vi "getCost.vi"(8 "error in (no error)":errorcluster, 11 "Espresso in":refnum<class "Espresso.lvclass">) -> (0 "error out":errorcluster, 2 "cost":dbl, 3 "Espresso out":refnum<class "Espresso.lvclass">)   [LabVIEW 2018, in "Espresso.lvclass"]
uses:
  Espresso.lvclass
  Beverage Class/Beverage.lvclass
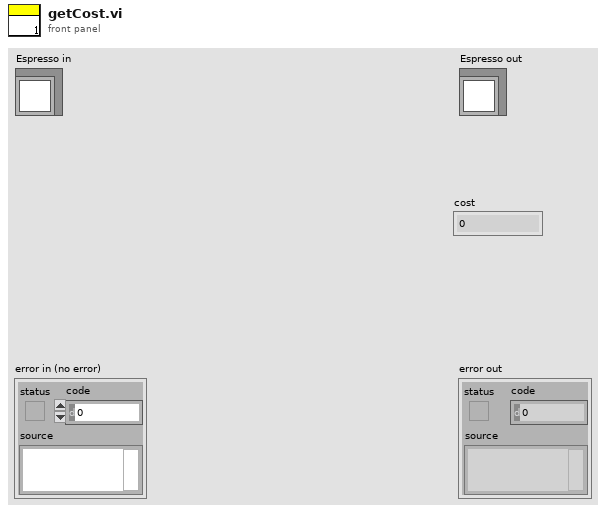
[diagram p1: front panel]
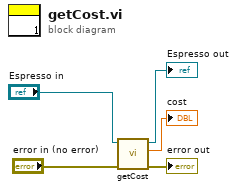
[diagram p0: block diagram]
diagram:
  n1 = call-parent "getCost.vi"("error in (no error)"="error in (no error)", "Beverage in"="Espresso in") -> ("error out"=→"error out":errorcluster, "cost"=→"cost":dbl, "Beverage out"=→"Espresso out":refnum<class "Espresso.lvclass">)  [unwired: 7 in]
